vi "DO Coil UI.vi"(8 "error in (no error)":errorcluster, 11 "Node Ptr":T3 format="%.0x") -> (0 "error out":errorcluster)   [LabVIEW 2015, in "Modbus Master System Explorer.lvlib"]
uses:
  Modbus Master System Explorer.lvlib
  <vilib>/NI Veristand/Custom Device API/Custom Device Item Ref.ctl
  SubVIs/Direction.ctl
  SubVIs/Radix.ctl
  <vilib>/NI VeriStand/Custom Device API/Custom Device API.lvlib
panel:
  in  "Radix":T1
  in  "Direction":T2
  out "Valid?":string
  in  "Address":u16
  in  "Header":cluster{"Section Name":string}={"Section Name"="Coil (Digital Out)"}
  in  "Description":string
  in  "Name":string
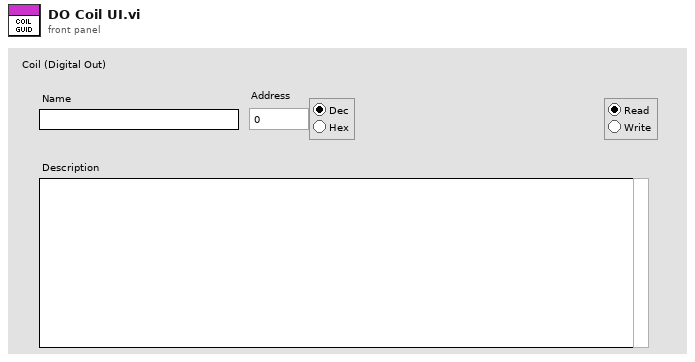
[diagram p1: front panel]
types:
  T1 = typedef "Modbus Master System Explorer.lvlib/Radix.ctl" = enum32{"Decimal", "Hexidecimal"}
  T2 = typedef "Modbus Master System Explorer.lvlib/Direction.ctl" = enum32{"Radio Selection 1", "Radio Selection 2"}
  T3 = typedef "Custom Device API.lvlib/Custom Device Item Ref.ctl" = u64
  T4 = typedef "Custom Device API.lvlib/Custom Device Commands.ctl" = enum16{"Default", "Item renamed", "Shutdown", "Dynamic button pressed"}
  T5 = typedef "Custom Device API.lvlib/Custom Device Item Info.ctl" = cluster{"Name":string, "Is Channel":bool, "GUID":string, "Is Waveform":bool}
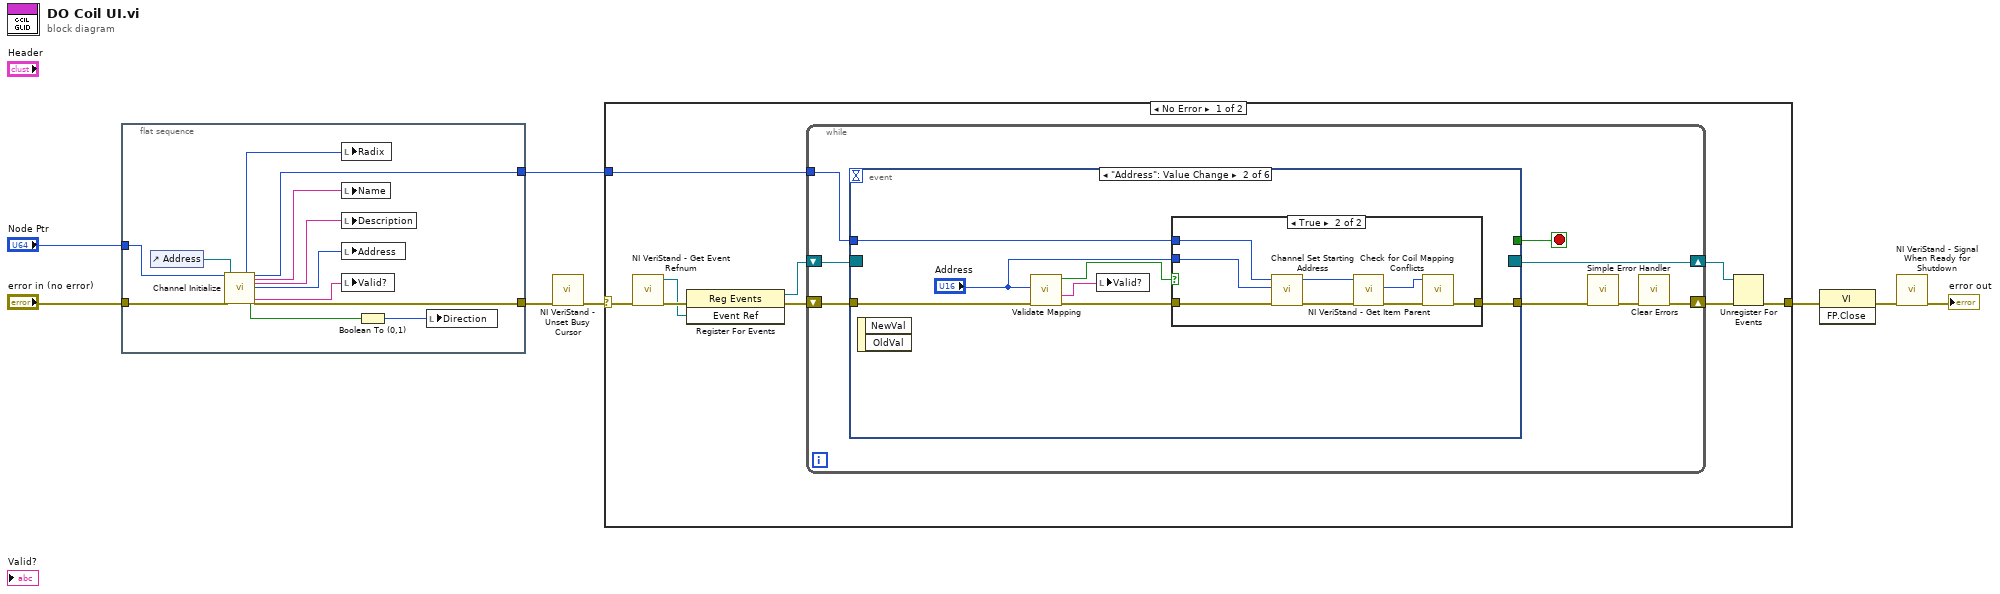
[diagram p0: block diagram]
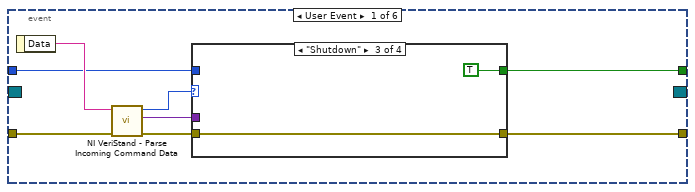
[diagram p2: hidden frame]
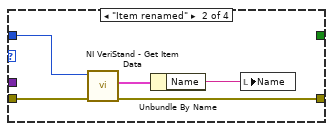
[diagram p4: hidden frame]
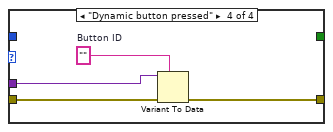
[diagram p5: hidden frame]
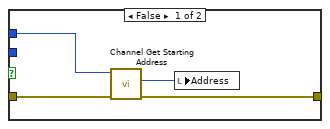
[diagram p6: hidden frame]
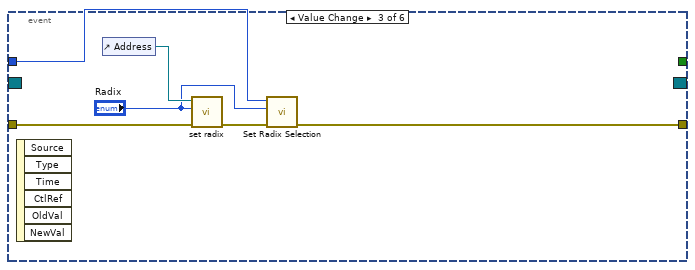
[diagram p7: hidden frame]
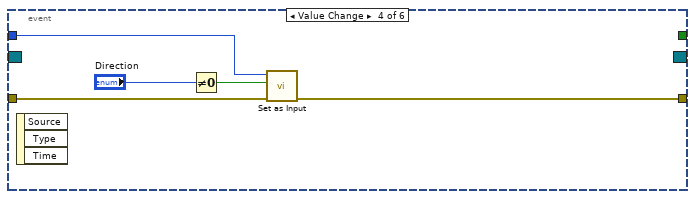
[diagram p8: hidden frame]
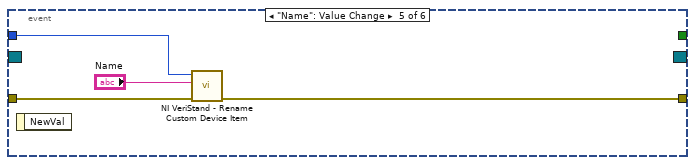
[diagram p9: hidden frame]
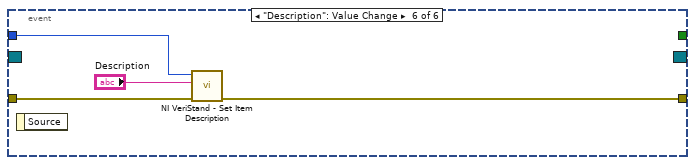
[diagram p10: hidden frame]
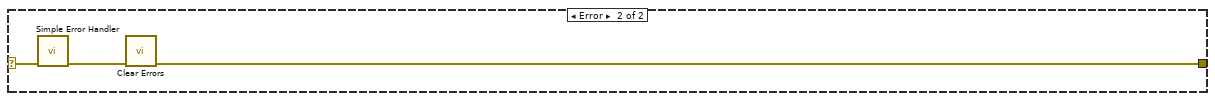
[diagram p11: hidden frame]
diagram:
  n1 = flat-sequence {
    tunnel: "Node Ptr" -> [w20]
    tunnel: [w11] -> w3
    tunnel: "error in (no error)" -> [w10]
    tunnel: [w9] -> w1
    frame #0 {
      n2 = control-ref of="Address"() -> (w19:refnum<vi>)
      n3 = call "Channel Initialize.vi"("Item Ref in"=w20, "error in (no error)"=w10, "Starting Address Ref in"=w19) -> ("Radix"=w18:T1, "input?"=w17:bool, "Channel Ref out"=w11:T3, "Name"=w13:string, "Description"=w12:string, "Starting Address"=w14:u16, "Status Message"=w15:string, "error out"=w9:errorcluster)  [unwired: 14 in, 3 out]
      n4 = local write "Radix"(w18) -> ()
      n5 = local write "Name"(w13) -> ()
      n6 = local write "Description"(w12) -> ()
      n7 = local write "Address"(w14) -> ()
      n8 = local write "Valid?"(w15) -> ()
      n9 = Boolean To (0,1)(Boolean=w17) -> (0, 1=w16:i16)
      n10 = local write "Direction"(w16) -> ()
    }
  }
  n11 = call <vilib>:"NI VeriStand - Unset Busy Cursor.vi"("error in (no error)"=w1) -> ("error out"=w5:errorcluster)  [unwired: 10 out]
  n12 = case shown="No Error" w5 {
    selector: w5 -> [w22 w98]
    tunnel: [w26 w96] -> w8
    tunnel: w3 -> [w23 _]
    frame No Error {
      n13 = call <vilib>:"NI VeriStand - Get Event Refnum.vi"("error in (no error)"=w22) -> ("error out"=w29:errorcluster, "Event Ref"=w21:refnum<user-event>)  [unwired: 9 out]
      n14 = register-events(error in=w29, w21) -> (reference out=w24:refnum<event-registration>, error out=w25:errorcluster)  [unwired: 1 in]
      n15 = while {
        tunnel: w23 -> [w33]
        shift-right: [w30] -> w27
        shift-left: w25 -> [w36]
        shift-right: [w37] -> w28
        shift-left: w24 -> [w35]
        stop <- w34 stop-if-true
        n16 = event shown="[1] \"Address\": Value Change" {
          selector: w35 -> [_ _ _ _ _ _]
          dyn-events: [_ _ _ _ _ _] -> w37
          timeout: _ -> [_ _ _ _ _ _]
          tunnel: w36 -> [w45 w63 w81 w86 w91 w94]
          tunnel: [w41 _ _ _ _ _] -> w34
          tunnel: [w40 w58 w79 w85 w90 w93] -> w32
          tunnel: w33 -> [w39 w61 w78 w87 w89 w95]
          event User Event {
            n17 = event-data() -> ("Data"=w44:string)  [unwired: 1 out]
            n18 = call <vilib>:"NI VeriStand - Parse Incoming Command Data.vi"("error in (no error)"=w45, "Incoming data"=w44) -> ("error out"=w43:errorcluster, "Outgoing data"=w38:variant, "Action"=w42:T4)  [unwired: 7 out]
            n19 = case shown="\"Shutdown\"" w42 {
              tunnel: w43 -> [w46 w51 w52 w57]
              tunnel: [_ _ TRUE _] -> w41
              tunnel: [w46 w48 w52 w54] -> w40
              tunnel: w39 -> [_ w50 _ _]
              tunnel: w38 -> [_ _ _ w56]
              frame "Default", Default {
              }
              frame "Item renamed" {
                n20 = call <vilib>:"NI VeriStand - Get Item Data.vi"("error in (no error)"=w51, "Item Ref in"=w50) -> ("error out"=w48:errorcluster, "Item Info"=w49:T5)  [unwired: 8 out]
                n21 = Unbundle By Name(w49) -> ("Name"=w47:string)
                n22 = local write "Name"(w47) -> ()
              }
              frame "Shutdown" {
              }
              frame "Dynamic button pressed" {
                w55 = ""  # Button ID
                n23 = Variant To Data(error in=w57, type=w55, Variant=w56) -> (error out=w54:errorcluster)  [unwired: 1 out]
              }
            }
          }
          event "Address": Value Change {
            n24 = event-data() -> ()  [unwired: 3 out]
            n25 = call "Validate Mapping.vi"("error in (no error)"=w63, "Mapping"="Address") -> ("error out"=w62:errorcluster, "Status Message"=w60:string, "Valid?"=w64:bool)  [unwired: 7 in]
            n26 = local write "Valid?"(w60) -> ()
            n27 = case shown="True" w64 {
              tunnel: w62 -> [w68 w74]
              tunnel: w61 -> [w65 w76]
              tunnel: "Address" -> [_ w75]
              tunnel: [w67 w69] -> w58
              frame False {
                n28 = call "Channel Get Starting Address.vi"("error in (no error)"=w68, "Item Ref in"=w65) -> ("error out"=w67:errorcluster, "Value"=w66:u16)  [unwired: 7 in, 1 out]
                n29 = local write "Address"(w66) -> ()
              }
              frame True {
                n30 = call "Channel Set Starting Address.vi"("error in (no error)"=w74, "Value"=w75, "Item Ref in"=w76) -> ("error out"=w71:errorcluster, "Item Ref out"=w73:T3)  [unwired: 7 in]
                n31 = call <vilib>:"NI VeriStand - Get Item Parent.vi"("error in (no error)"=w71, "Item Ref in"=w73) -> ("error out"=w70:errorcluster, "Parent Ref"=w72:T3)  [unwired: 6 in, 2 out]
                n32 = call "Check for Coil Mapping Conflicts.vi"("error in (no error)"=w70, "Coiil Group Ref in"=w72) -> ("error out"=w69:errorcluster)  [unwired: 6 in, 3 out]
              }
            }
          }
          event Value Change {
            n33 = event-data() -> ()  [unwired: 7 out]
            n34 = control-ref of="Address"() -> (w82:refnum<vi>)
            n35 = call "set radix.vi"("error in (no error)"=w81, "Radix"="Radix", "Digital in"=w82) -> ("error out"=w80:errorcluster)  [unwired: 8 in]
            n36 = call "Set Radix Selection.vi"("error in (no error)"=w80, "Radix"="Radix", "Item Ref in"=w78) -> ("error out"=w79:errorcluster)  [unwired: 7 in, 1 out]
          }
          event Value Change {
            n37 = event-data() -> ()  [unwired: 4 out]
            n38 = Not Equal To 0?(x="Direction") -> (x != 0?=w83:bool)
            n39 = call "Set as Input.vi"("error in (no error)"=w86, "Direction"=w83, "Channel Ref in"=w87) -> ("error out"=w85:errorcluster)  [unwired: 7 in, 1 out]
          }
          event "Name": Value Change {
            n40 = event-data() -> ()  [unwired: 2 out]
            n41 = call <vilib>:"NI VeriStand - Rename Custom Device Item.vi"("error in (no error)"=w91, "New Name"="Name", "Item Ref in"=w89) -> ("error out"=w90:errorcluster)  [unwired: 1 in, 7 out]
          }
          event "Description": Value Change {
            n42 = event-data() -> ()  [unwired: 2 out]
            n43 = call <vilib>:"NI VeriStand - Set Item Description.vi"("error in (no error)"=w94, "Description"="Description", "Item Ref in"=w95) -> ("error out"=w93:errorcluster)  [unwired: 8 out]
          }
        }
        n44 = call <vilib>:"Simple Error Handler.vi"("error in (no error)"=w32) -> ("error out"=w31:errorcluster)  [unwired: 1 in, 7 out]
        n45 = call <vilib>:"Clear Errors.vi"("error in (no error)"=w31) -> ("error out"=w30:errorcluster)  [unwired: 1 in, 5 out]
      }
      n46 = Unregister For Events(event registration refnum=w28, error in=w27) -> (error out=w26:errorcluster)
    }
    frame Error {
      n47 = call <vilib>:"Simple Error Handler.vi"("error in (no error)"=w98) -> ("error out"=w97:errorcluster)  [unwired: 1 in, 7 out]
      n48 = call <vilib>:"Clear Errors.vi"("error in (no error)"=w97) -> ("error out"=w96:errorcluster)  [unwired: 1 in, 5 out]
    }
  }
  n49 = invoke class="VI" method="FP.Close"(error in=w8) -> (error out=w7:errorcluster)  [unwired: 2 in, 2 out]
  n50 = call <vilib>:"NI VeriStand - Signal When Ready for Shutdown.vi"("error in (no error)"=w7) -> ("error out"=→"error out":errorcluster)  [unwired: 10 out]
